vi "trash_move_Sort Loaded Plugins.vi"(3 "Plugin Info":T14(array[cluster]) {"Plugin Connections"."Plugin Info"."Node Status"."Monitor Doubles"."4" format="%#_9g"; "Plugin Connections"."Plugin Info"."Node Status"."Monitor Doubles"."3" format="%#_9g"; "Plugin Connections"."Plugin Info"."Node Status"."Monitor Doubles"."2" format="%#_9g"; "Plugin Connections"."Plugin Info"."Node Status"."Monitor Doubles"."1" format="%#_9g"; "Plugin Connections"."Plugin Info"."Node Status"."Timing Statistics (us)"."Period"."Avg" format="%_6g"}) -> (5 "Sorted Plugin Info":T14(array[cluster]) {"Plugin Connections"."Plugin Info"."Node Status"."Monitor Doubles"."4" format="%#_9g"; "Plugin Connections"."Plugin Info"."Node Status"."Monitor Doubles"."3" format="%#_9g"; "Plugin Connections"."Plugin Info"."Node Status"."Monitor Doubles"."2" format="%#_9g"; "Plugin Connections"."Plugin Info"."Node Status"."Monitor Doubles"."1" format="%#_9g"; "Plugin Connections"."Plugin Info"."Node Status"."Timing Statistics (us)"."Period"."Avg" format="%_6g"})   [LabVIEW 2021]
uses:
  Typedef/trash_Plugin Connections.ctl
  <vilib>/gRPC/LabVIEW gRPC Library/Shared/grpcId.ctl
  Typedef/PluginInfo.ctl
  Typedef/trash_Version.ctl
  <vilib>/CIF Foundation/CIF Core/CIFCore/Common/Typedef/gRPC Reported Plugin Status.ctl
  <vilib>/CIF Foundation/CIF Core/CIFCore/Common/Typedef/Plugin State.ctl
  <vilib>/CIF Foundation/CIF Core/CIFCore/Common/Typedef/Timing Statistics.ctl
  <vilib>/CIF Foundation/CIF Core/CIFCore/Common/Typedef/Timing Stats Base.ctl
  <vilib>/CIF Foundation/CIF Core/CIFCore/Common/Typedef/FIFO Statistics.ctl
  <vilib>/CIF Foundation/CIF Core/CIFCore/Common/Typedef/Simple Error.ctl
  <vilib>/CIF Foundation/CIF Core/CIFCore/Common/Typedef/Monitor Doubles.ctl
  <vilib>/CIF Foundation/CIF Core/CIFCore/Common/Typedef/Monitor U64.ctl
  <vilib>/CIF Foundation/CIF Core/CIFCore/Common/Typedef/Monitor I64.ctl
  5a2b8e69-9079-4bc9-912e-d849fb448030.vi
  <vilib>/Comparison/Less/Less Functor/Less Functor.lvclass
  CIF_Manager_UI.lvclass/CIF_Manager_UI.ctl
  <vilib>/gRPC/LabVIEW gRPC Library/grpc-lvsupport-release.lvlib
  <vilib>/CIF Foundation/CIF Core/CIFCore/Common/CIFCoreCommon.lvlib
  CIF_Manager_UI.lvclass
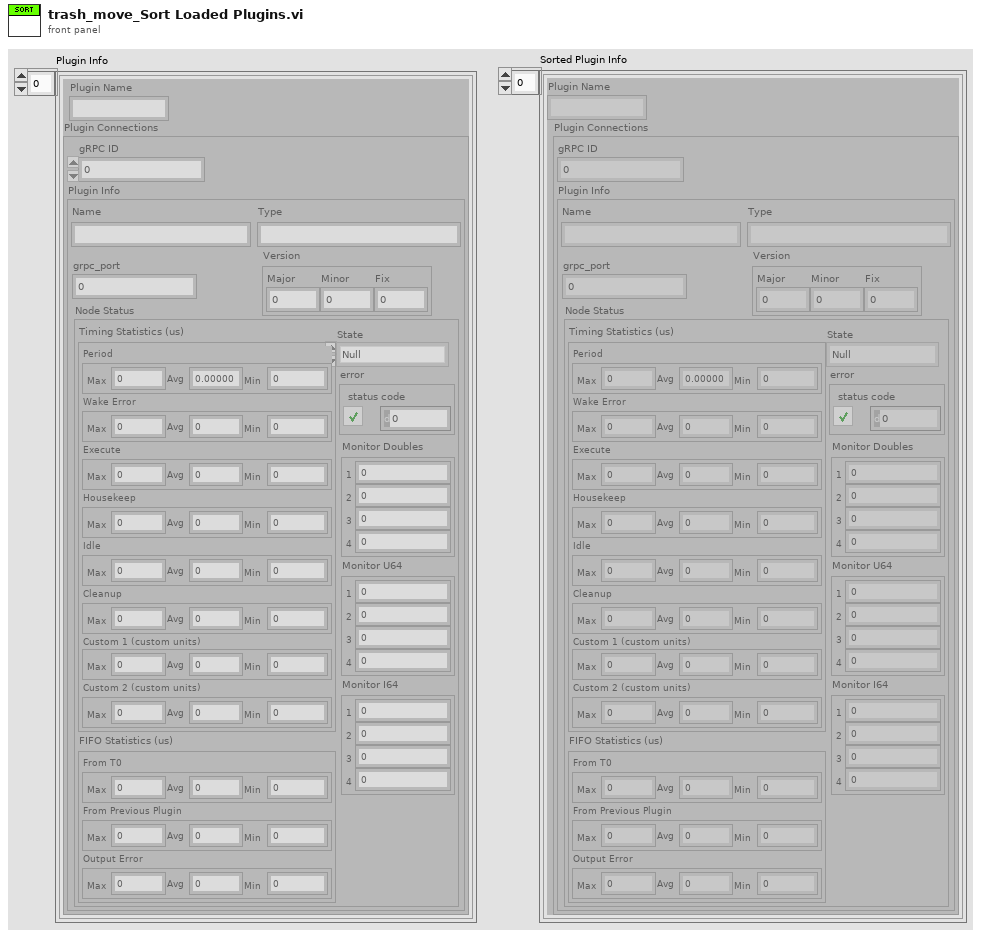
[diagram p1: front panel]
types:
  T1 = typedef "trash_Plugin Connections.ctl" = cluster{"gRPC ID":T2, "Plugin Info":T3}
  T2 = typedef "grpc-lvsupport-release.lvlib/grpcId.ctl" = u64
  T3 = typedef "CIF_Manager_UI.lvclass/PluginInfo.ctl" = cluster{"Name":string, "Type":string, "grpc_port":i32, "Version":T4, "Node Status":T5}
  T4 = typedef "trash_Version.ctl" = cluster{"Major":i32, "Minor":i32, "Fix":i32}
  T5 = typedef "CIFCoreCommon.lvlib/gRPC Reported Plugin Status.ctl" = cluster{"State":T6, "Timing Statistics (us)":T7, "FIFO Statistics (us)":T9, "error":T10, "Monitor Doubles":T11, "Monitor U64":T12, "Monitor I64":T13}
  T6 = typedef "CIFCoreCommon.lvlib/Plugin State.ctl" = enum32{"Null", "Creating", "Listening", "Running", "CleaningUp", "Destroying"}
  T7 = typedef "CIFCoreCommon.lvlib/Timing Statistics.ctl" = cluster{"Period":T8, "Wake Error":T8, "Execute":T8, "Housekeep":T8, "Idle":T8, "Cleanup":T8, "Custom 1 (custom units)":T8, "Custom 2 (custom units)":T8}
  T8 = typedef "CIFCoreCommon.lvlib/Timing Stats Base.ctl" = cluster{"Max":i64, "Avg":dbl, "Min":i64}
  T9 = typedef "CIFCoreCommon.lvlib/FIFO Statistics.ctl" = cluster{"From T0":T8, "From Previous Plugin":T8, "Output Error":T8}
  T10 = typedef "CIFCoreCommon.lvlib/Simple Error.ctl" = cluster{"status":bool, "code":i32}
  T11 = typedef "CIFCoreCommon.lvlib/Monitor Doubles.ctl" = cluster{"1":dbl, "2":dbl, "3":dbl, "4":dbl}
  T12 = typedef "CIFCoreCommon.lvlib/Monitor U64.ctl" = cluster{"1":u64, "2":u64, "3":u64, "4":u64}
  T13 = typedef "CIFCoreCommon.lvlib/Monitor I64.ctl" = cluster{"1":i64, "2":i64, "3":i64, "4":i64}
  T14 = cluster{"Plugin Name":string, "Plugin Connections":T1}[]
  T15 = cluster{string, "Plugin Info":cluster{"Plugin Name":string, "Plugin Connections":T1}}
  T16 = cluster{string, "Plugin Info":cluster{"Plugin Name":string, "Plugin Connections":T1}}[]
  T17 = cluster{"Plugin Name":string, "Plugin Connections":T1}
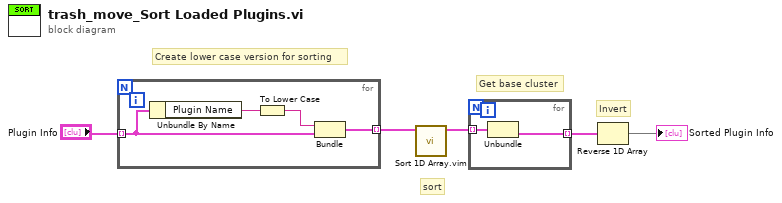
[diagram p0: block diagram]
diagram:
  # "Invert"
  # "Get base cluster"
  # "sort"
  # "Create lower case version for sorting"
  n1 = for {
    tunnel: "Plugin Info" -> [w7] mode=indexing
    tunnel: [w9] -> w5 mode=indexing
    n2 = Unbundle By Name(w7) -> ("Plugin Name"=w8:string)
    n3 = To Lower Case(string=w8) -> (all lower case string=w6:string)
    n4 = Bundle(w6, "Plugin Info"=w7) -> (w9:T15)  [unwired: 1 in]
  }
  n5 = call "Sort 1D Array.vim"("unsorted array"=w5) -> ("sorted array"=w4:T16)  [unwired: 10 in]
  n6 = for {
    tunnel: w4 -> [w11] mode=indexing
    tunnel: [w10] -> w2 mode=indexing
    n7 = Unbundle(w11) -> ("Plugin Info"=w10:T17)  [unwired: 1 out]
  }
  n8 = Reverse 1D Array(array=w2) -> (reversed array=→"Sorted Plugin Info":T14)
